vi "JFTBwavegeneration2 (1).vi"() -> ()   [LabVIEW 2023]
uses:
  <vilib>/Analysis/5stat.llb/RMS (DBL).vi
  <vilib>/measure/maspectr.llb/FFT Power Spectrum and PSD for N Chan.vi
  <vilib>/measure/NI_MAPro.lvlib
  <vilib>/Analysis/NI_AALPro.lvlib
panel:
  in  "High Pass Cut-Off (Hz)":dbl=5000.0 caption="Lower Cut-Off"
  in  "Lower Cut-Off (Hz)":dbl=200.0 caption="Lower Cut-Off"
  in  "High Pass Filter":bool
  in  "Lo-Pass Filter":bool
  in  "Record Sound":bool
  in  "Duration Control (sec)":dbl
  out "Max SPL (NOT in dB - For Comparison Purposes ONLY)":dbl
  out "FFT of Recorded Sound":cluster{"f0":dbl, "df":dbl, "magnitude":dbl[]}[](graph)
  out "Recorded Waveform":dynamicdata(graph)
  in  "Play Sound":bool
  in  "End Program":bool
  in  "8th":dbl
  in  "7th":dbl
  in  "6th":dbl
  in  "5th":dbl
  in  "4th":dbl
  in  "3rd":dbl
  in  "2nd":dbl
  in  "1st":dbl
  in  "Fund.\n Frequeny":dbl
  in  "Amplitude":dbl[](array[slide]) scale=0.0..1000.0
  out "Generated Sound FFT":cluster{"f0":dbl, "df":dbl, "magnitude":dbl[]}[](graph)
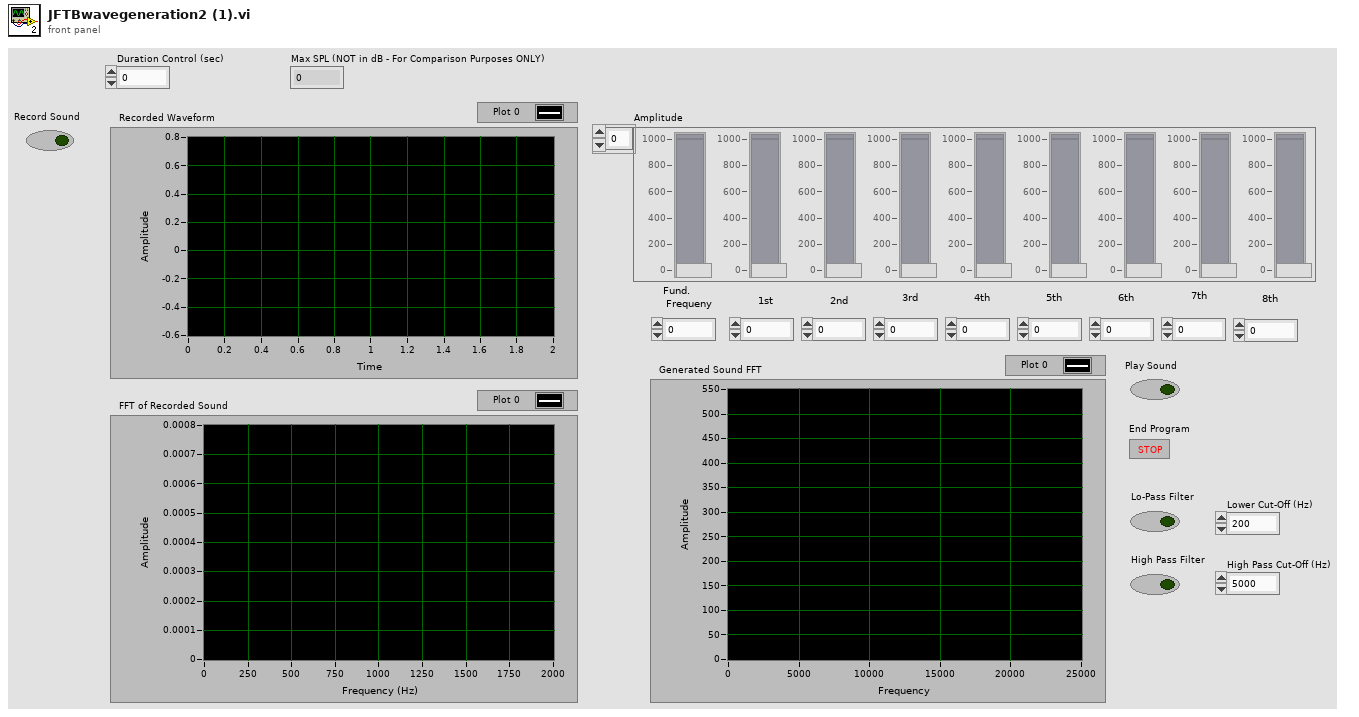
[diagram p1: front panel]
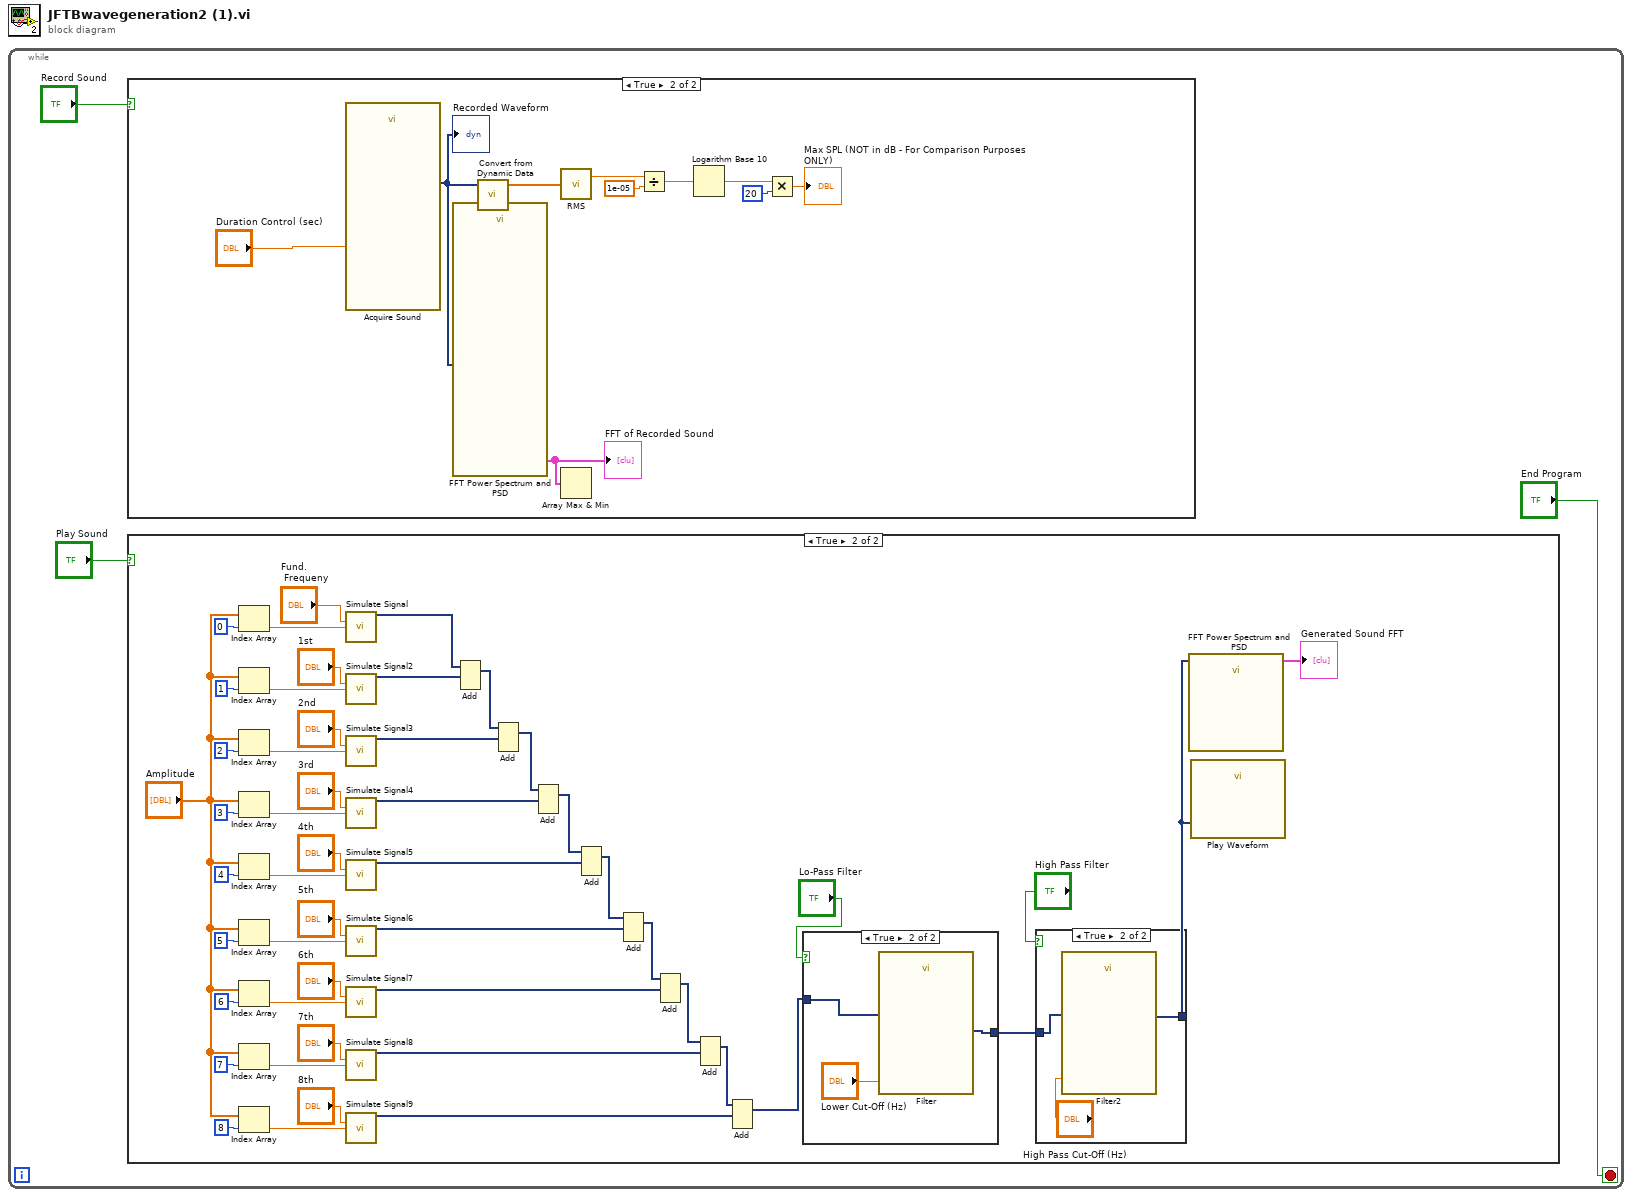
[diagram p0: block diagram]
diagram:
  n1 = while {
    stop <- "End Program" stop-if-true
    n2 = case shown="True" "Record Sound" {
      frame False {
      }
      frame True {
        n3 = call "Acquire Sound"("Duration (s)"="Duration Control (sec)") -> ("Data"=w11:dynamicdata)  [unwired: 17 in, 1 out]
        "Recorded Waveform" <- w11
        n4 = call-poly <vilib>:"FFT Power Spectrum and PSD.vi"("time signals"=w11) -> ("Power Spectrum / PSD"=w13:cluster{"f0":dbl, "df":dbl, "magnitude":dbl[]}[])  [unwired: 7 in, 3 out]
        "FFT of Recorded Sound" <- w13
        n5 = call "Convert from Dynamic Data"("Dynamic Data Type"=w11) -> ("Array"=w10:dbl[])  [unwired: 3 in]
        n6 = call-poly <vilib>:"RMS.vi"("X"=w10) -> ("rms value"=w9:dbl)  [unwired: 1 out]
        n7 = Array Max & Min(array=w13) -> ()  [unwired: 4 out]
        n8 = Divide(x=w9, y=1e-05) -> (x/y=w7:dbl)
        n9 = Logarithm Base 10(1:w7) -> (0:w5:dbl)
        n10 = Multiply(x=w5, y=20) -> (x*y=→"Max SPL (NOT in dB - For Comparison Purposes ONLY)":dbl)
      }
    }
    n11 = case shown="True" "Play Sound" {
      frame False {
      }
      frame True {
        n12 = Index Array(array="Amplitude", index=0) -> (element=w51:dbl)
        n13 = Index Array(array="Amplitude", index=1) -> (element=w52:dbl)
        n14 = Index Array(array="Amplitude", index=2) -> (element=w50:dbl)
        n15 = Index Array(array="Amplitude", index=3) -> (element=w47:dbl)
        n16 = Index Array(array="Amplitude", index=4) -> (element=w43:dbl)
        n17 = Index Array(array="Amplitude", index=5) -> (element=w36:dbl)
        n18 = Index Array(array="Amplitude", index=6) -> (element=w33:dbl)
        n19 = Index Array(array="Amplitude", index=7) -> (element=w28:dbl)
        n20 = Index Array(array="Amplitude", index=8) -> (element=w24:dbl)
        n21 = call "Simulate Signal"("Frequency"="Fund.\n Frequeny", "Amplitude"=w51) -> ("Sine"=w63:dynamicdata)  [unwired: 12 in, 1 out]
        n22 = call "Simulate Signal2"("Frequency"="1st", "Amplitude"=w52) -> ("Sine"=w62:dynamicdata)  [unwired: 12 in, 1 out]
        n23 = call "Simulate Signal3"("Frequency"="2nd", "Amplitude"=w50) -> ("Sine"=w60:dynamicdata)  [unwired: 12 in, 1 out]
        n24 = call "Simulate Signal4"("Frequency"="3rd", "Amplitude"=w47) -> ("Sine"=w45:dynamicdata)  [unwired: 12 in, 1 out]
        n25 = call "Simulate Signal5"("Frequency"="4th", "Amplitude"=w43) -> ("Sine"=w42:dynamicdata)  [unwired: 12 in, 1 out]
        n26 = call "Simulate Signal6"("Frequency"="5th", "Amplitude"=w36) -> ("Sine"=w38:dynamicdata)  [unwired: 12 in, 1 out]
        n27 = call "Simulate Signal7"("Frequency"="6th", "Amplitude"=w33) -> ("Sine"=w32:dynamicdata)  [unwired: 12 in, 1 out]
        n28 = call "Simulate Signal8"("Frequency"="7th", "Amplitude"=w28) -> ("Sine"=w26:dynamicdata)  [unwired: 12 in, 1 out]
        n29 = call "Simulate Signal9"("Frequency"="8th", "Amplitude"=w24) -> ("Sine"=w19:dynamicdata)  [unwired: 12 in, 1 out]
        n30 = Add(1:w62, 2:w63) -> (0:w61:dynamicdata)  [unwired: 1 in, 1 out]
        n31 = Add(1:w60, 2:w61) -> (0:w46:dynamicdata)  [unwired: 1 in, 1 out]
        n32 = Add(1:w45, 2:w46) -> (0:w41:dynamicdata)  [unwired: 1 in, 1 out]
        n33 = Add(1:w42, 2:w41) -> (0:w37:dynamicdata)  [unwired: 1 in, 1 out]
        n34 = Add(1:w38, 2:w37) -> (0:w31:dynamicdata)  [unwired: 1 in, 1 out]
        n35 = Add(1:w32, 2:w31) -> (0:w25:dynamicdata)  [unwired: 1 in, 1 out]
        n36 = Add(1:w26, 2:w25) -> (0:w20:dynamicdata)  [unwired: 1 in, 1 out]
        n37 = Add(1:w19, 2:w20) -> (0:w18:dynamicdata)  [unwired: 1 in, 1 out]
        n38 = case shown="True" "Lo-Pass Filter" {
          tunnel: w18 -> [w68 w71]
          tunnel: [w68 w70] -> w15
          frame False {
          }
          frame True {
            n39 = call "Filter"("Lower Cut-Off"="Lower Cut-Off (Hz)", "Signal"=w71) -> ("Filtered Signal"=w70:dynamicdata)  [unwired: 8 in, 1 out]
          }
        }
        n40 = case shown="True" "High Pass Filter" {
          tunnel: w15 -> [w64 w67]
          tunnel: [w64 w66] -> w14
          frame False {
          }
          frame True {
            n41 = call "Filter2"("Lower Cut-Off"="High Pass Cut-Off (Hz)", "Signal"=w67) -> ("Filtered Signal"=w66:dynamicdata)  [unwired: 8 in, 1 out]
          }
        }
        n42 = call-poly <vilib>:"FFT Power Spectrum and PSD.vi"("time signals"=w14) -> ("Power Spectrum / PSD"=→"Generated Sound FFT":cluster{"f0":dbl, "df":dbl, "magnitude":dbl[]}[])  [unwired: 7 in, 3 out]
        n43 = call "Play Waveform"("Data"=w14) -> ()  [unwired: 18 in, 1 out]
      }
    }
  }
